vi "Read Actors VI Ref.vi"(8 "error in (no error)":errorcluster, 11 "Superior Actor in":refnum<class "Root Actor.lvclass">) -> (0 "error out":errorcluster, 2 "Actors VI Ref":refnum<vi>[](array[refnum]), 3 "Superior Actor out":refnum<class "Root Actor.lvclass">)   [LabVIEW 2019, in "Root Actor.lvclass"]
uses:
  Root Actor.lvclass
  Messenger/Mail Strategy/Mail Strategy.lvclass
  System Actor/System Actor.lvclass
  Root Actor.lvclass/Root Actor.ctl
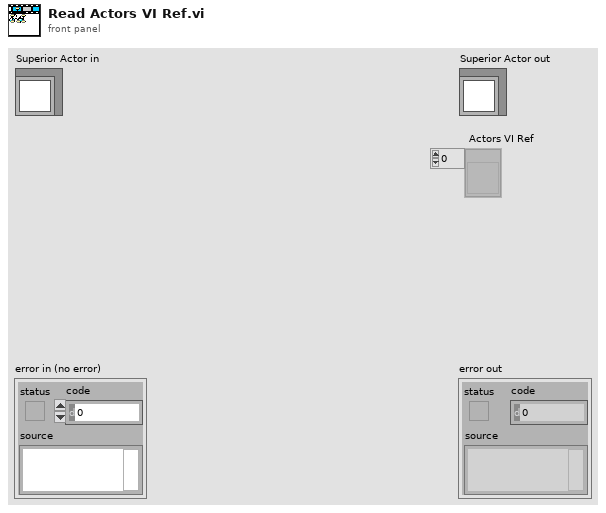
[diagram p1: front panel]
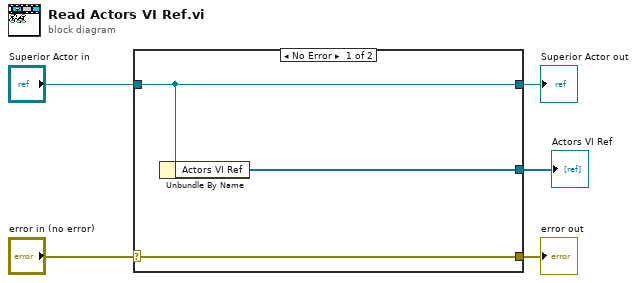
[diagram p0: block diagram]
diagram:
  n1 = case shown="No Error" "error in (no error)" {
    selector: "error in (no error)" -> [w8 w9]
    tunnel: [w8 w9] -> w4
    tunnel: [w7 w10] -> w2
    tunnel: "Superior Actor in" -> [w7 w10]
    tunnel: [w6 _] -> w1
    frame No Error {
      n2 = Unbundle By Name(w7) -> ("Actors VI Ref"=w6:refnum<vi>[])
    }
    frame Error {
    }
  }
  "error out" <- w4
  "Superior Actor out" <- w2
  "Actors VI Ref" <- w1
